vi "DRC Read Sample.vi"(2 "Point #":i32, 3 "Instrument Address":refnum<visa-resource-name>) -> (0 "Stop":bool, 1 "Output":dbl[](array[numeric]) format="%.2f")   [LabVIEW 2019]
doc: "This VI reads the sample output of the Lakeshore DRC 93C or 82C temperature controller. The output is an array consisting of the single reading. The input is the numeric GPIB address.\nScott Hannahs, F. Bitter National Magnet Lab, 1993"
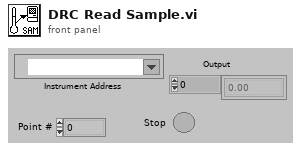
[diagram p1: front panel]
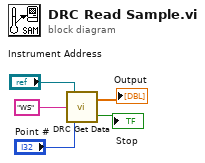
[diagram p0: block diagram]
diagram:
  n1 = call "DRC Get Data.vi"("Point #"="Point #", "Command String"="WS", "Instrument Address"="Instrument Address") -> ("Stop"=→"Stop":bool, "Output"=→"Output":dbl[])
